vi "send pre-tomo on to thor.vi"(8 "error in (no error)":errorcluster, 10 "FPS":dbl, 11 "Tomo in":refnum<class "Tomo.lvclass">) -> (0 "error out":errorcluster, 3 "Tomo out":refnum<class "Tomo.lvclass">)   [LabVIEW 2012, in "Tomo.lvclass"]
uses:
  Tomo.lvclass
  <vilib>/Distrio/Murmex/Murmex/update_cluster.ctl
  <vilib>/Distrio/Murmex/GenericMessage/GenericMessage.lvclass
  Tomo.lvclass/Tomo.ctl
  <vilib>/Distrio/Murmex/Message/Add or replace parameter.vi
  <vilib>/Distrio/Murmex/Murmex/Murmex.lvclass
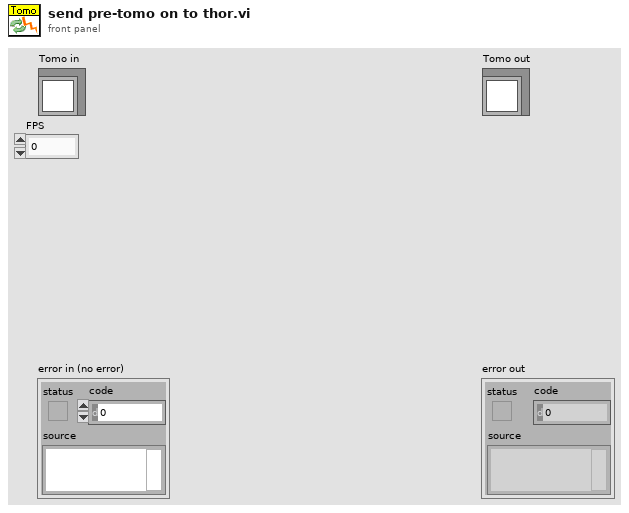
[diagram p1: front panel]
types:
  T1 = typedef "Murmex.lvlib/Murmex.lvclass/update_cluster.ctl" = cluster{"target ID":string, "key chains":string[], "values":variant[]}
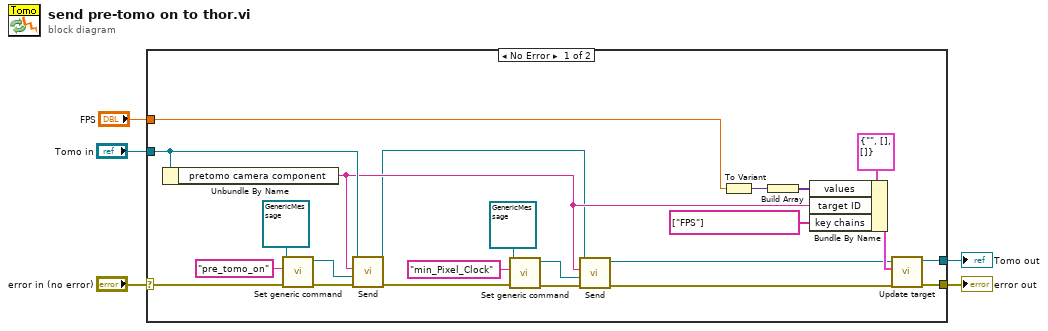
[diagram p0: block diagram]
diagram:
  n1 = case shown="No Error" "error in (no error)" {
    selector: "error in (no error)" -> [w23 w30]
    tunnel: [w19 w30] -> w4
    tunnel: [w17 w29] -> w1
    tunnel: "Tomo in" -> [w24 w29]
    tunnel: "FPS" -> [w15 _]
    frame No Error {
      n2 = Unbundle By Name(w24) -> ("pretomo camera component"=w8:string)
      n3 = call <vilib>:"Set generic command.vi"("error in (no error)"=w23, "generic command"="pre_tomo_on", "GenericMessage in"=refnum<class "GenericMessage.lvclass"> refnum ("Distrio Murmex 1.1:GenericMessage")) -> ("error out"=w26:errorcluster, "GenericMessage out"=w25:refnum<class "GenericMessage.lvclass">)  [unwired: 7 in]
      n4 = call <vilib>:"Send.vi"("error in (no error)"=w26, "Message"=w25, "recipient"=w8, "Murmex in"=w24) -> ("error out"=w10:errorcluster, "Murmex out"=w7:refnum<class "Tomo.lvclass">)  [unwired: 6 in]
      n5 = call <vilib>:"Set generic command.vi"("error in (no error)"=w10, "generic command"="min_Pixel_Clock", "GenericMessage in"=refnum<class "GenericMessage.lvclass"> refnum ("Distrio Murmex 1.1:GenericMessage")) -> ("error out"=w13:errorcluster, "GenericMessage out"=w14:refnum<class "GenericMessage.lvclass">)  [unwired: 7 in]
      n6 = call <vilib>:"Send.vi"("error in (no error)"=w13, "Message"=w14, "recipient"=w8, "Murmex in"=w7) -> ("error out"=w9:errorcluster, "Murmex out"=w6:refnum<class "Tomo.lvclass">)  [unwired: 6 in]
      n7 = To Variant(anything=w15) -> (Variant=w21:variant)
      n8 = Build Array(w21) -> (w18:variant[])
      n9 = Bundle By Name(cluster=T1 {"target ID"="", "key chains"=[], "values"=[]} ("update cluster"), "values"=w18, "target ID"=w8, "key chains"=string[] ["FPS"]) -> (w20:T1)
      n10 = call <vilib>:"Update target.vi"("error in (no error)"=w9, "update cluster"=w20, "MurmexBase in"=w6) -> ("error out"=w19:errorcluster, "MurmexBase out"=w17:refnum<class "Tomo.lvclass">)  [unwired: 7 in]
    }
    frame Error {
    }
  }
  "error out" <- w4
  "Tomo out" <- w1
